vi "Get 2400 output.vi"(5 "Check For SCPI Errors? (T)":bool=TRUE, 8 "error in (no error)":errorcluster, 11 "Resource In":refnum<visa-resource-name>) -> (0 "Output State":T1, 3 "Resource Out (dupl)":refnum<visa-resource-name>)   [LabVIEW 2019, in "Get value.lvlib"]
uses:
  Get value.lvlib
  lib/Keithley 622x/Typedefs/KE622x -- On Off Control.ctl
  lib/Keithley 622x/Keithley 622x.lvlib
panel:
  out "error out":errorcluster
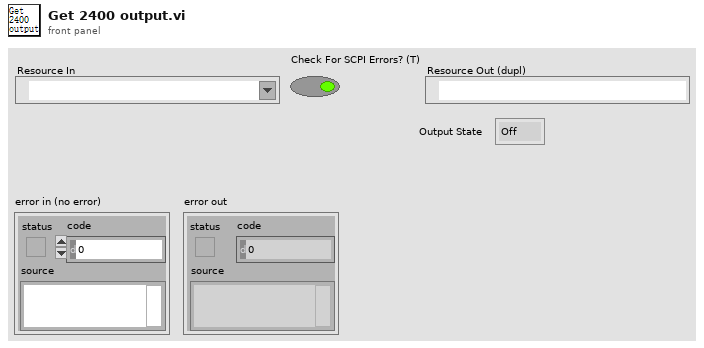
[diagram p1: front panel]
types:
  T1 = typedef "Keithley 622x.lvlib/KE622x -- On Off Control.ctl" = enum16{"Off", "On"}
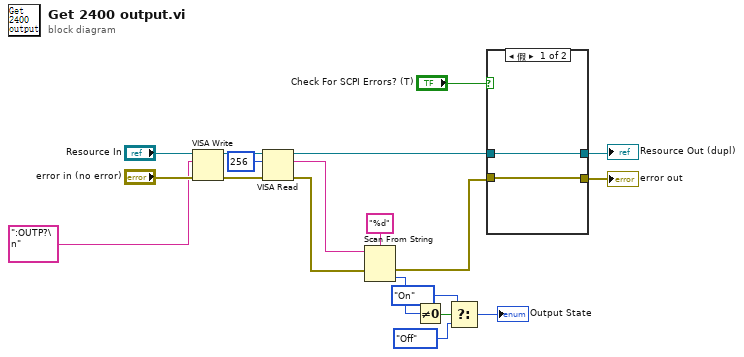
[diagram p0: block diagram]
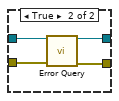
[diagram p2: hidden frame]
diagram:
  n1 = VISA Write(VISA resource name="Resource In", write buffer=":OUTP?\n" ("format string"), error in (no error)="error in (no error)") -> (VISA resource name out=w13:refnum<visa-resource-name>, error out=w12:errorcluster)  [unwired: 1 out]
  n2 = VISA Read(VISA resource name=w13, byte count=u32 256, error in (no error)=w12) -> (VISA resource name out=w7:refnum<visa-resource-name>, read buffer=w6:string, error out=w10:errorcluster)  [unwired: 1 out]
  n3 = Scan From String(format string="%d", input string=w6, error in=w10) -> (error out=w8:errorcluster, output 1=w5:i32)  [unwired: 2 in, 2 out]
  n4 = Not Equal To 0?(x=w5) -> (x != 0?=w4:bool)
  n5 = Select(t=KE622x_--_On_Off_Control."On", s=w4, f=KE622x_--_On_Off_Control."Off" ("Output State")) -> (s? t:f=→"Output State":T1)
  n6 = case shown="假" "Check For SCPI Errors? (T)" {
    tunnel: w7 -> [w21 w25]
    tunnel: w8 -> [w20 w24]
    tunnel: [w20 w23] -> w15
    tunnel: [w21 w22] -> w16
    frame False {
    }
    frame True {
      n7 = call "Error Query.vi"("VISA Resource In"=w25, "error in (no error)"=w24) -> ("VISA Resource Out (dupl)"=w22:refnum<visa-resource-name>, "error out"=w23:errorcluster)  [unwired: 10 in, 2 out]
    }
  }
  "Resource Out (dupl)" <- w16
  "error out" <- w15
